vi "LEDActionsController.vi"(11 "Action":T1) -> (3 "PWM Output":dbl)   [LabVIEW 2018]
uses:
  Actions.ctl
  <vilib>/Rock Robotics/Network Tables/NT Write Number.vi
panel:
  in  "Numeric":dbl=0.57 format="%#_13g"
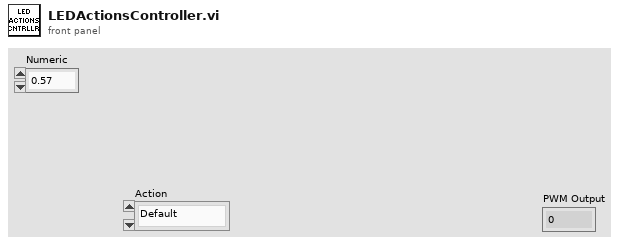
[diagram p1: front panel]
types:
  T1 = typedef "Actions.ctl" = enum16{"Default", "Hatch Triggered", "Lost Vision", "Auto Aiming", "Party Mode", "Has Hatch"}
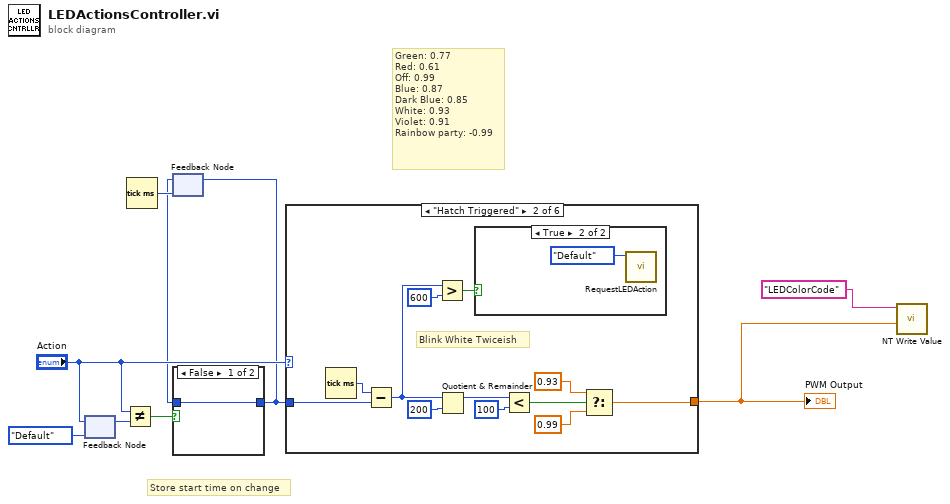
[diagram p0: block diagram]
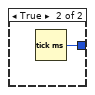
[diagram p2: hidden frame]
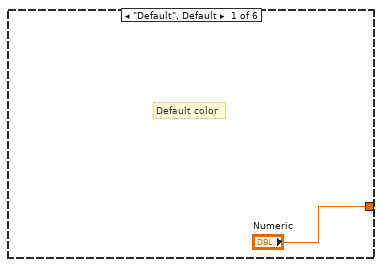
[diagram p3: hidden frame]
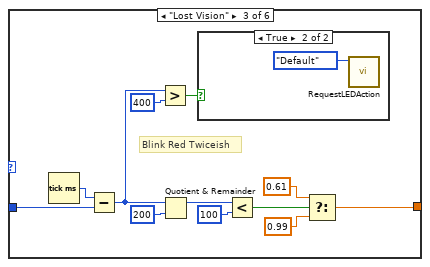
[diagram p5: hidden frame]
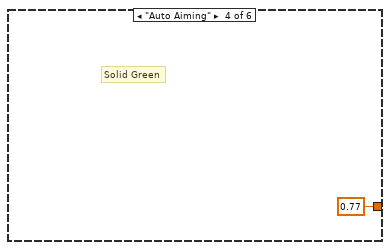
[diagram p7: hidden frame]
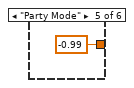
[diagram p8: hidden frame]
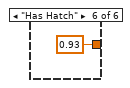
[diagram p9: hidden frame]
diagram:
  # "Green: 0.77\nRed: 0.61\nOff: 0.99\nBlue: 0.87\nDark Blue: 0.85\nWhite: 0.93\nViolet: 0.91\nRainbow party: -0.99"
  # "Store start time on change"
  n1 = feedback-in #1("Action") -> ()
  n2 = feedback #1(Actions."Default" ("Action")) -> (w7:T1)
  n3 = Not Equal?(x="Action", y=w7) -> (x != y?=w4:bool)
  n4 = Tick Count (ms)() -> (millisecond timer value=w9:u32)
  n5 = feedback #2(w9) -> (w5:u32)
  n6 = case shown="False" w4 {
    tunnel: [w10 w11] -> w3
    tunnel: w5 -> [w10 _]
    frame False {
    }
    frame True {
      n7 = Tick Count (ms)() -> (millisecond timer value=w11:u32)
    }
  }
  n8 = feedback-in #2(w3) -> ()
  n9 = case shown="\"Hatch Triggered\"" "Action" {
    tunnel: ["Numeric" w24 w37 0.77 ("f") -0.99 ("f") 0.93 ("f")] -> w1
    tunnel: w3 -> [_ w23 w36 _ _ _]
    frame "Default", Default {
      # "Default color"
    }
    frame "Hatch Triggered" {
      # "Blink White Twiceish"
      n10 = Tick Count (ms)() -> (millisecond timer value=w22:u32)
      n11 = Subtract(x=w22, y=w23) -> (x-y=w19:u32)
      n12 = Greater?(x=w19, y=u32 600) -> (0:w16:bool)
      n13 = Quotient & Remainder(x=w19, y=u32 200) -> (x-y*floor(x/y)=w15:u32)  [unwired: 1 out]
      n14 = case shown="True" w16 {
        frame False {
        }
        frame True {
          n15 = call "RequestLEDAction.vi"("Action"=Actions."Default") -> ()  [unwired: 11 in]
        }
      }
      n16 = Less?(x=w15, y=u32 100) -> (x < y?=w17:bool)
      n17 = Select(t=0.93, s=w17, f=0.99) -> (s? t:f=w24:dbl)
    }
    frame "Lost Vision" {
      # "Blink Red Twiceish"
      n18 = Tick Count (ms)() -> (millisecond timer value=w35:u32)
      n19 = Subtract(x=w35, y=w36) -> (x-y=w32:u32)
      n20 = Greater?(x=w32, y=u32 400) -> (0:w29:bool)
      n21 = Quotient & Remainder(x=w32, y=u32 200) -> (x-y*floor(x/y)=w28:u32)  [unwired: 1 out]
      n22 = case shown="True" w29 {
        frame False {
        }
        frame True {
          n23 = call "RequestLEDAction.vi"("Action"=Actions."Default") -> ()  [unwired: 11 in]
        }
      }
      n24 = Less?(x=w28, y=u32 100) -> (x < y?=w30:bool)
      n25 = Select(t=0.61, s=w30, f=0.99) -> (s? t:f=w37:dbl)
    }
    frame "Auto Aiming" {
      # "Solid Green"
    }
    frame "Party Mode" {
    }
    frame "Has Hatch" {
    }
  }
  "PWM Output" <- w1
  n26 = call-poly <vilib>:"NT Write Value.vi"("Numeric"=w1, "Name"="LEDColorCode") -> ()  [unwired: 9 in, 1 out]
